vi "Load BG Image from File by Name.vi"(8 "error in (no error)":errorcluster, 10 "BG Image FIle Name":string, 11 "HIJ Vision Camera App in":refnum<class "HIJ Vision Camera App.lvclass">) -> (0 "error out":errorcluster, 3 "HIJ Vision Camera App out":refnum<class "HIJ Vision Camera App.lvclass">)   [LabVIEW 2020, in "HIJ Vision Camera App.lvlib" / "HIJ Vision Camera App.lvclass"]
uses:
  HIJ Vision Camera App.lvclass
  C:/Users/AlexK/work/LabVIEW Programme/POLARIS CAM Log Abw und E/Submodules/HIJ Vision/Application Base Actors/HIJ Vision Application/HIJ Vision Application/HIJ Vision Application.lvclass
  HIJ Vision Application/HIJ Vision Application/HIJ Vision Application.lvclass/HIJ Vision Application.ctl
  HIJ Vision Application/HIJ Vision Application/Read WorkDir.vi
  HIJ Vision Camera App.lvclass/HIJ Vision Camera App.ctl
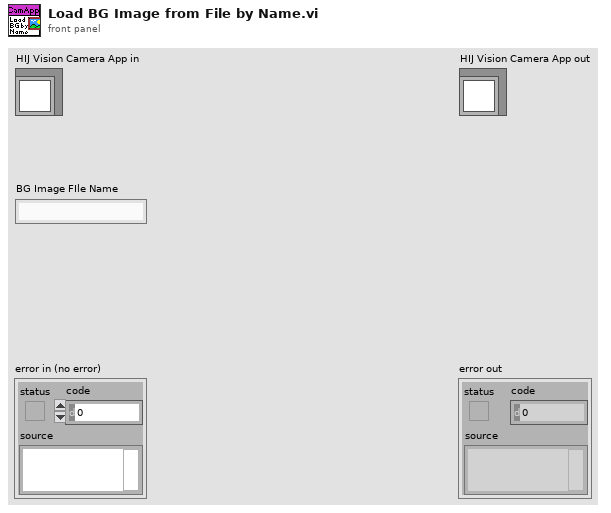
[diagram p1: front panel]
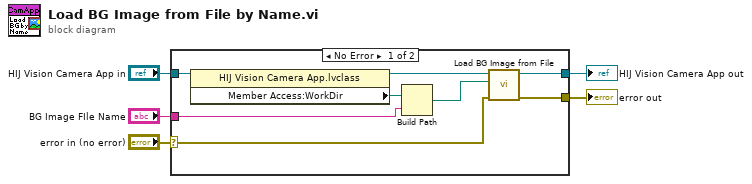
[diagram p0: block diagram]
diagram:
  n1 = case shown="No Error" "error in (no error)" {
    selector: "error in (no error)" -> [w7 w15]
    tunnel: [w6 w15] -> w4
    tunnel: [w9 w14] -> w2
    tunnel: "HIJ Vision Camera App in" -> [w13 w14]
    tunnel: "BG Image FIle Name" -> [w10 _]
    frame No Error {
      n2 = property class="HIJ Vision Camera App.lvclass"(reference=w13) -> (reference out=w12:refnum<class "HIJ Vision Camera App.lvclass">, "Member Access:WorkDir"=w11:path)  [unwired: 1 in, 1 out]
      n3 = Build Path(base path=w11, name or relative path=w10) -> (appended path=w8:path)
      n4 = call-dynamic "Load BG Image from File.vi"("error in (no error)"=w7, "BG Image Path"=w8, "HIJ Vision Camera App in"=w12) -> ("error out"=w6:errorcluster, "HIJ Vision Camera App out"=w9:refnum<class "HIJ Vision Camera App.lvclass">)  [unwired: 7 in]
    }
    frame Error {
    }
  }
  "error out" <- w4
  "HIJ Vision Camera App out" <- w2
